vi "Fc_Get_TRACEDATA.vi"(6 "Start+timeout?":bool, 8 "error in (no error)":errorcluster, 11 "Class TCP in":T1) -> (0 "error out":errorcluster, 3 "Class TCP out":T1)   [LabVIEW 2022 SP3]
doc: "This function calls the microcontroller to obtain the signal data and stores them at the time of the request, into the \"Signals_value_Array\" variable."
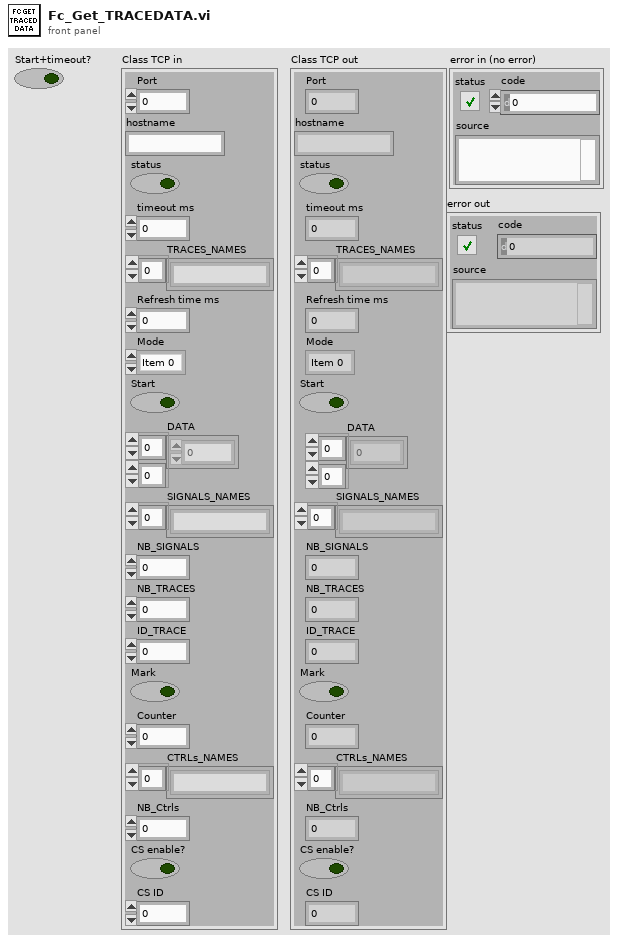
[diagram p1: front panel]
types:
  T1 = cluster{"Port":i32, "hostname":string, "status":bool, "timeout ms":i32, "TRACES_NAMES":string[], "Refresh time ms":i32, "Mode":enum32{"Item 0", "Item 1"}, "Start":bool, "DATA":sgl[][], "SIGNALS_NAMES":string[], "NB_SIGNALS":i32, "NB_TRACES":i32, "ID_TRACE":i32, "Mark":bool, "Counter":i32, "CTRLs_NAMES":string[], "NB_Ctrls":i32, "CS enable?":bool, "CS ID":i32}
  T2 = cluster{"TRACE_SIZE":i32, "CS_ID":i32, "TRACE ID":i32, "CMD":i32, "DATA(M)":i32}
  T3 = cluster{"timeout ms":i32, "remote port":u16, "Address":string}
  T4 = cluster{"SIZE":i32, " TRACE DATA":sgl[], "TRACE_SIZE":i32, "NB_TRACES":i32, "NB_TRACED_SIGNALS":i32, "NAMES TRACED SIGNALS":string[], "NAMES TRACES":string[], "CS STATUS":i32, "NB_CSs":i32, "NAMES CSs":string[], "DATA (M)":sgl[], "CMD":i32}
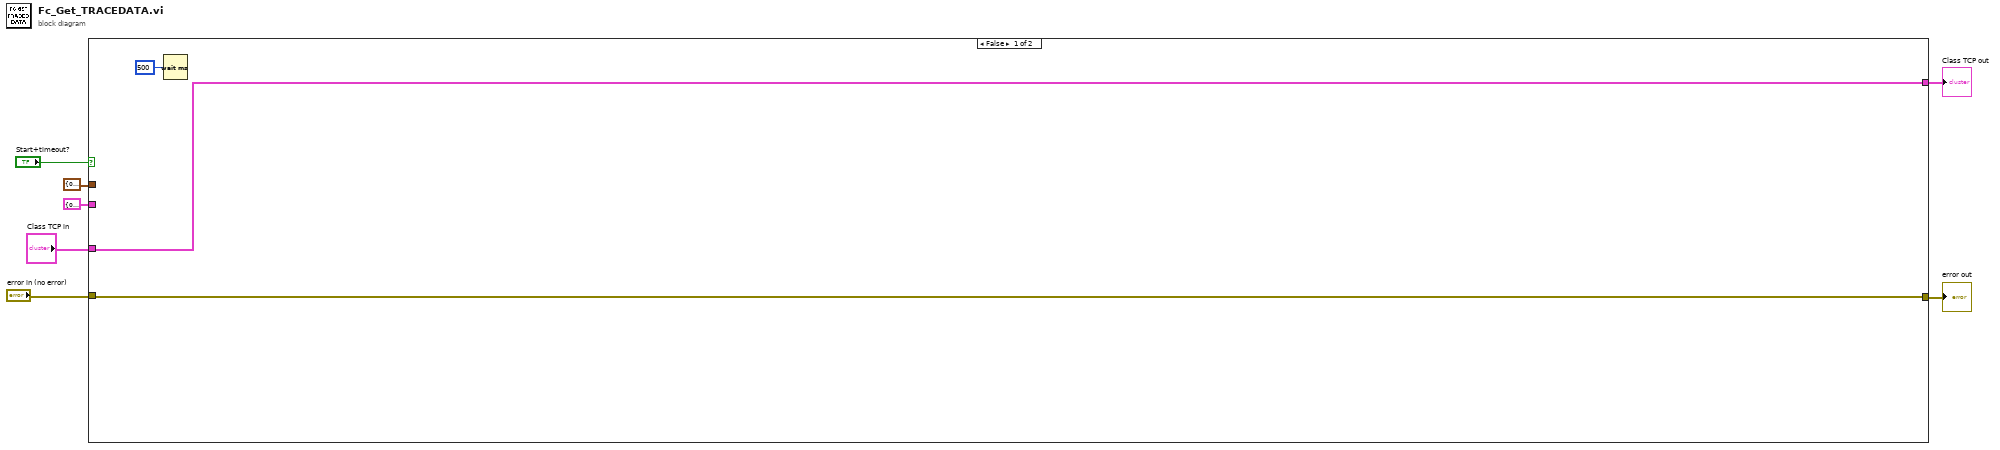
[diagram p0: block diagram]
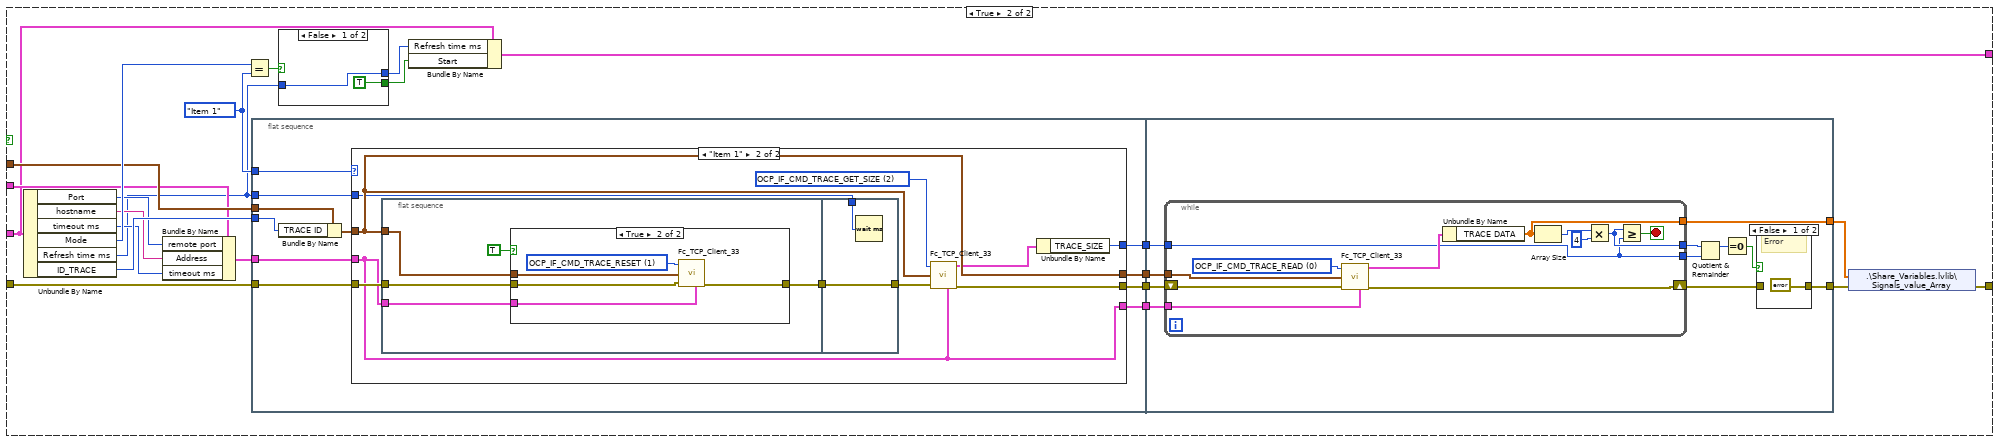
[diagram p2: hidden frame]
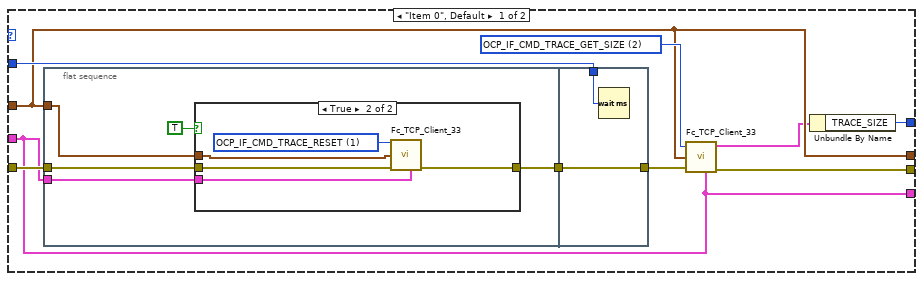
[diagram p3: hidden frame]
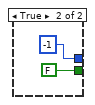
[diagram p7: hidden frame]
diagram:
  n1 = case shown="False" "Start+timeout?" {
    tunnel: "Class TCP in" -> [w10 w22]
    tunnel: [w10 w29] -> w5
    tunnel: T2 {"TRACE_SIZE"=0, "CS_ID"=0, "TRACE ID"=0, "CMD"=0, "DATA(M)"=0} ("Input Cluster") -> [_ w24]
    tunnel: T3 {"timeout ms"=0, "remote port"=0, "Address"=""} ("Comunication Cluster") -> [_ w23]
    tunnel: "error in (no error)" -> [w9 w20]
    tunnel: [w9 w19] -> w1
    frame False {
      n2 = Wait (ms)(milliseconds to wait=u32 500) -> ()  [unwired: 1 out]
    }
    frame True {
      w21 = enum32{"Item 0", "Item 1"}."Item 1" ("Mode")
      n3 = Unbundle By Name(w22) -> ("Port"=w28:i32, "hostname"=w27:string, "timeout ms"=w17:i32, "Mode"=w33:enum32{"Item 0", "Item 1"}, "Refresh time ms"=w11:i32, "ID_TRACE"=w30:i32)
      n4 = Bundle By Name(cluster=w23, "remote port"=w28, "Address"=w27, "timeout ms"=w17) -> (w26:T3)
      n5 = Equal?(x=w33, y=w21) -> (x = y?=w32:bool)
      n6 = flat-sequence {
        tunnel: w26 -> [w42]
        tunnel: w24 -> [w38]
        tunnel: w30 -> [w44]
        tunnel: [w43] -> w16
        tunnel: [w41] -> w15
        tunnel: [w40] -> w14
        tunnel: w21 -> [w39]
        tunnel: w20 -> [w36]
        tunnel: [w35] -> w13
        tunnel: w11 -> [w34]
        tunnel: w16 -> [w99]
        tunnel: w15 -> [w101]
        tunnel: w14 -> [w100]
        tunnel: [w98] -> w18
        tunnel: w13 -> [w97]
        tunnel: [w91] -> w25
        frame #0 {
          n7 = Bundle By Name(cluster=w38, "TRACE ID"=w44) -> (w37:T2)
          n8 = case shown="\"Item 1\"" w39 {
            tunnel: [w50 w76] -> w43
            tunnel: w42 -> [w49 w74]
            tunnel: [w49 w74] -> w41
            tunnel: [w45 w73] -> w40
            tunnel: w37 -> [w50 w76]
            tunnel: w36 -> [w53 w77]
            tunnel: [w47 w71] -> w35
            tunnel: w34 -> [w52 w69]
            frame "Item 0", Default {
              w51 = 2 items=["OCP_IF_CMD_TRACE_READ", "OCP_IF_CMD_TRACE_RESET", "OCP_IF_CMD_TRACE_GET_SIZE", "OCP_IF_CMD_TRACE_SET_SIZE", "OCP_IF_CMD_TRACE_GET_NUMBER_SIGNALS", "OCP_IF_CMD_TRACE_GET_SIGNALS_NAMES", "OCP_IF_CMD_TRACE_GET_NUMBER_TRACES", "OCP_IF_CMD_TRACE_GET_TRACES_NAMES", "OCP_IF_CMD_TRACE_GET_ADDRESS", "OCP_IF_CMD_CS_STATUS", "OCP_IF_CMD_CS_ENABLE", "OCP_IF_CMD_CS_DISABLE", "OCP_IF_CMD_CS_CONTROLLER_IF", "OCP_IF_CMD_CS_HARDWARE_IF", "OCP_IF_CMD_CS_GET_NUMBER_CONTROLLERS", "OCP_IF_CMD_CS_GET_CONTROLLERS_NAMES", "OCP_IF_CMD_PLATFORM_ID", "OCP_IF_CMD_PLATFORM_IF", "OCP_IF_CMD_OPIL_UPDATE_MEASUREMENTS", "OCP_IF_CMD_OPIL_UPDATE_SIM_DATA", "OCP_IF_CMD_OPIL_RUN_CONTROL", "OCP_IF_CMD_OPIL_INITIALIZE_CONTROL", "OCP_IF_CMD_OPIL_GET_CONTROL", "OCP_IF_CMD_OPIL_GET_CONTROLLER_DATA", "OCP_IF_CMD_END"] ("CMD")
              n9 = flat-sequence {
                tunnel: w53 -> [w59]
                tunnel: w50 -> [w58]
                tunnel: w49 -> [w56]
                tunnel: [w57] -> w54
                tunnel: [w67] -> w46
                tunnel: w54 -> [w67]
                tunnel: w52 -> [w66]
                frame #0 {
                  n10 = case shown="True" TRUE {
                    tunnel: w59 -> [w60 w64]
                    tunnel: w58 -> [_ w63]
                    tunnel: [w60 w62] -> w57
                    tunnel: w56 -> [_ w61]
                    frame False {
                    }
                    frame True {
                      w65 = 1 items=["OCP_IF_CMD_TRACE_READ", "OCP_IF_CMD_TRACE_RESET", "OCP_IF_CMD_TRACE_GET_SIZE", "OCP_IF_CMD_TRACE_SET_SIZE", "OCP_IF_CMD_TRACE_GET_NUMBER_SIGNALS", "OCP_IF_CMD_TRACE_GET_SIGNALS_NAMES", "OCP_IF_CMD_TRACE_GET_NUMBER_TRACES", "OCP_IF_CMD_TRACE_GET_TRACES_NAMES", "OCP_IF_CMD_TRACE_GET_ADDRESS", "OCP_IF_CMD_CS_STATUS", "OCP_IF_CMD_CS_ENABLE", "OCP_IF_CMD_CS_DISABLE", "OCP_IF_CMD_CS_CONTROLLER_IF", "OCP_IF_CMD_CS_HARDWARE_IF", "OCP_IF_CMD_CS_GET_NUMBER_CONTROLLERS", "OCP_IF_CMD_CS_GET_CONTROLLERS_NAMES", "OCP_IF_CMD_PLATFORM_ID", "OCP_IF_CMD_PLATFORM_IF", "OCP_IF_CMD_OPIL_UPDATE_MEASUREMENTS", "OCP_IF_CMD_OPIL_UPDATE_SIM_DATA", "OCP_IF_CMD_OPIL_RUN_CONTROL", "OCP_IF_CMD_OPIL_INITIALIZE_CONTROL", "OCP_IF_CMD_OPIL_GET_CONTROL", "OCP_IF_CMD_OPIL_GET_CONTROLLER_DATA", "OCP_IF_CMD_END"] ("CMD")
                      n11 = call "Fc_TCP_Client_33.vi"("CMD"=w65, "Input Cluster"=w63, "error in (no error)"=w64, "Comunication Cluster"=w61) -> ("error out"=w62:errorcluster)  [unwired: 4 in, 2 out]
                    }
                  }
                }
                frame #1 {
                  n12 = Wait (ms)(milliseconds to wait=w66) -> ()  [unwired: 1 out]
                }
              }
              n13 = call "Fc_TCP_Client_33.vi"("CMD"=w51, "Input Cluster"=w50, "error in (no error)"=w46, "Comunication Cluster"=w49) -> ("Output cluster"=w48:T4, "error out"=w45:errorcluster)  [unwired: 4 in, 1 out]
              n14 = Unbundle By Name(w48) -> ("TRACE_SIZE"=w47:i32)
            }
            frame "Item 1" {
              w68 = 2 items=["OCP_IF_CMD_TRACE_READ", "OCP_IF_CMD_TRACE_RESET", "OCP_IF_CMD_TRACE_GET_SIZE", "OCP_IF_CMD_TRACE_SET_SIZE", "OCP_IF_CMD_TRACE_GET_NUMBER_SIGNALS", "OCP_IF_CMD_TRACE_GET_SIGNALS_NAMES", "OCP_IF_CMD_TRACE_GET_NUMBER_TRACES", "OCP_IF_CMD_TRACE_GET_TRACES_NAMES", "OCP_IF_CMD_TRACE_GET_ADDRESS", "OCP_IF_CMD_CS_STATUS", "OCP_IF_CMD_CS_ENABLE", "OCP_IF_CMD_CS_DISABLE", "OCP_IF_CMD_CS_CONTROLLER_IF", "OCP_IF_CMD_CS_HARDWARE_IF", "OCP_IF_CMD_CS_GET_NUMBER_CONTROLLERS", "OCP_IF_CMD_CS_GET_CONTROLLERS_NAMES", "OCP_IF_CMD_PLATFORM_ID", "OCP_IF_CMD_PLATFORM_IF", "OCP_IF_CMD_OPIL_UPDATE_MEASUREMENTS", "OCP_IF_CMD_OPIL_UPDATE_SIM_DATA", "OCP_IF_CMD_OPIL_RUN_CONTROL", "OCP_IF_CMD_OPIL_INITIALIZE_CONTROL", "OCP_IF_CMD_OPIL_GET_CONTROL", "OCP_IF_CMD_OPIL_GET_CONTROLLER_DATA", "OCP_IF_CMD_END"] ("CMD")
              n15 = flat-sequence {
                tunnel: w77 -> [w82]
                tunnel: w76 -> [w81]
                tunnel: w74 -> [w79]
                tunnel: [w80] -> w70
                tunnel: [w90] -> w75
                tunnel: w70 -> [w90]
                tunnel: w69 -> [w89]
                frame #0 {
                  n16 = case shown="True" TRUE {
                    tunnel: w82 -> [w83 w87]
                    tunnel: w81 -> [_ w86]
                    tunnel: [w83 w85] -> w80
                    tunnel: w79 -> [_ w84]
                    frame False {
                    }
                    frame True {
                      w88 = 1 items=["OCP_IF_CMD_TRACE_READ", "OCP_IF_CMD_TRACE_RESET", "OCP_IF_CMD_TRACE_GET_SIZE", "OCP_IF_CMD_TRACE_SET_SIZE", "OCP_IF_CMD_TRACE_GET_NUMBER_SIGNALS", "OCP_IF_CMD_TRACE_GET_SIGNALS_NAMES", "OCP_IF_CMD_TRACE_GET_NUMBER_TRACES", "OCP_IF_CMD_TRACE_GET_TRACES_NAMES", "OCP_IF_CMD_TRACE_GET_ADDRESS", "OCP_IF_CMD_CS_STATUS", "OCP_IF_CMD_CS_ENABLE", "OCP_IF_CMD_CS_DISABLE", "OCP_IF_CMD_CS_CONTROLLER_IF", "OCP_IF_CMD_CS_HARDWARE_IF", "OCP_IF_CMD_CS_GET_NUMBER_CONTROLLERS", "OCP_IF_CMD_CS_GET_CONTROLLERS_NAMES", "OCP_IF_CMD_PLATFORM_ID", "OCP_IF_CMD_PLATFORM_IF", "OCP_IF_CMD_OPIL_UPDATE_MEASUREMENTS", "OCP_IF_CMD_OPIL_UPDATE_SIM_DATA", "OCP_IF_CMD_OPIL_RUN_CONTROL", "OCP_IF_CMD_OPIL_INITIALIZE_CONTROL", "OCP_IF_CMD_OPIL_GET_CONTROL", "OCP_IF_CMD_OPIL_GET_CONTROLLER_DATA", "OCP_IF_CMD_END"] ("CMD")
                      n17 = call "Fc_TCP_Client_33.vi"("CMD"=w88, "Input Cluster"=w86, "error in (no error)"=w87, "Comunication Cluster"=w84) -> ("error out"=w85:errorcluster)  [unwired: 4 in, 2 out]
                    }
                  }
                }
                frame #1 {
                  n18 = Wait (ms)(milliseconds to wait=w89) -> ()  [unwired: 1 out]
                }
              }
              n19 = call "Fc_TCP_Client_33.vi"("CMD"=w68, "Input Cluster"=w76, "error in (no error)"=w75, "Comunication Cluster"=w74) -> ("Output cluster"=w72:T4, "error out"=w73:errorcluster)  [unwired: 4 in, 1 out]
              n20 = Unbundle By Name(w72) -> ("TRACE_SIZE"=w71:i32)
            }
          }
        }
        frame #1 {
          n21 = while {
            tunnel: w101 -> [w113]
            tunnel: w99 -> [w111]
            tunnel: [w109] -> w98
            shift-right: [w115] -> w92
            shift-left: w100 -> [w112]
            tunnel: w97 -> [w104]
            tunnel: [w105] -> w94
            tunnel: [w104] -> w93
            stop <- w106 stop-if-true
            w114 = 0 items=["OCP_IF_CMD_TRACE_READ", "OCP_IF_CMD_TRACE_RESET", "OCP_IF_CMD_TRACE_GET_SIZE", "OCP_IF_CMD_TRACE_SET_SIZE", "OCP_IF_CMD_TRACE_GET_NUMBER_SIGNALS", "OCP_IF_CMD_TRACE_GET_SIGNALS_NAMES", "OCP_IF_CMD_TRACE_GET_NUMBER_TRACES", "OCP_IF_CMD_TRACE_GET_TRACES_NAMES", "OCP_IF_CMD_TRACE_GET_ADDRESS", "OCP_IF_CMD_CS_STATUS", "OCP_IF_CMD_CS_ENABLE", "OCP_IF_CMD_CS_DISABLE", "OCP_IF_CMD_CS_CONTROLLER_IF", "OCP_IF_CMD_CS_HARDWARE_IF", "OCP_IF_CMD_CS_GET_NUMBER_CONTROLLERS", "OCP_IF_CMD_CS_GET_CONTROLLERS_NAMES", "OCP_IF_CMD_PLATFORM_ID", "OCP_IF_CMD_PLATFORM_IF", "OCP_IF_CMD_OPIL_UPDATE_MEASUREMENTS", "OCP_IF_CMD_OPIL_UPDATE_SIM_DATA", "OCP_IF_CMD_OPIL_RUN_CONTROL", "OCP_IF_CMD_OPIL_INITIALIZE_CONTROL", "OCP_IF_CMD_OPIL_GET_CONTROL", "OCP_IF_CMD_OPIL_GET_CONTROLLER_DATA", "OCP_IF_CMD_END"] ("CMD")
            n22 = call "Fc_TCP_Client_33.vi"("CMD"=w114, "Input Cluster"=w111, "error in (no error)"=w112, "Comunication Cluster"=w113) -> ("Output cluster"=w110:T4, "error out"=w115:errorcluster)  [unwired: 4 in, 1 out]
            n23 = Unbundle By Name(w110) -> ("TRACE DATA"=w109:sgl[])
            n24 = Array Size(array=w109) -> (size(s)=w108:i32)
            n25 = Multiply(x=w108, y=4) -> (x*y=w105:i32)
            n26 = Greater Or Equal?(x=w105, y=w104) -> (x >= y?=w106:bool)
          }
          n27 = Quotient & Remainder(x=w94, y=w93) -> (x-y*floor(x/y)=w96:i32)  [unwired: 1 out]
          n28 = Equal To 0?(x=w96) -> (x = 0?=w95:bool)
          n29 = case shown="False" w95 {
            tunnel: w92 -> [_ w103]
            tunnel: [errorcluster {"status"=TRUE, "code"=5001, "source"="Not match value of Trace_data_size and Trace_Size"} ("error out") w103] -> w91
            frame False {
              # "Error"
            }
            frame True {
            }
          }
        }
      }
      n30 = case shown="False" w32 {
        tunnel: [TRUE FALSE] -> w31
        tunnel: [w116 i8 -1 ("t")] -> w12
        tunnel: w11 -> [w116 _]
        frame False {
        }
        frame True {
        }
      }
      n31 = Bundle By Name(cluster=w22, "Refresh time ms"=w12, "Start"=w31) -> (w29:T1)
      n32 = shared-variable ".\\Share_Variables.lvlib\\Signals_value_Array"(w18, error in=w25) -> (error out=w19:errorcluster)
    }
  }
  "Class TCP out" <- w5
  "error out" <- w1
